vi "Create Session.vi"(8 "error in (no error)":errorcluster) -> (0 "error out":errorcluster, 3 "Session Handle":refnum<data-value>)   [LabVIEW 2020, in "G-Embedded-Python-Interpreter-Toolkit.lvlib"]
uses:
  G-Embedded-Python-Interpreter-Toolkit.lvlib
  bin/gepit.cp310.32.dll
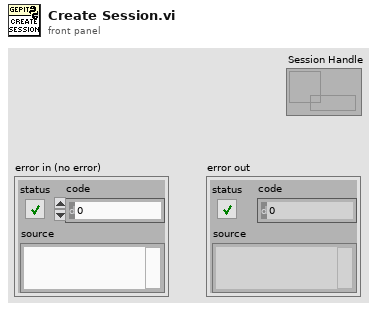
[diagram p1: front panel]
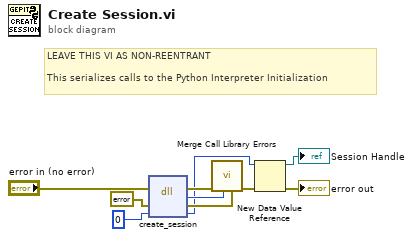
[diagram p0: block diagram]
diagram:
  # "LEAVE THIS VI AS NON-REENTRANT\n\nThis serializes calls to the Python Interpreter Initialization"
  n1 = dll-call lib="C:/serenial/libraries/g-embedded-python-interpreter-toolkit/LabVIEW/bin/gepit.cp310.32.dll" fn="create_session"(error in="error in (no error)", "Error"=errorcluster {"status"=FALSE, "code"=0, "source"=""} ("error constant"), "Session"=u64 0) -> (error out=w8:errorcluster, "return type"=w7:i32, "Error"=w6:errorcluster, "Session"=w3:u64)  [unwired: 2 in, 1 out]
  n2 = call "Merge Call Library Errors.vi"("Call Library Error"=w6, "Return Value"=w7, "error in"=w8) -> ("error out"=w4:errorcluster)  [unwired: 8 in]
  n3 = New Data Value Reference(data value=w3, error in=w4) -> (data value reference=→"Session Handle":refnum<data-value>, error out=→"error out":errorcluster)
